vi "剔除拟合空白数据.vi"(2 "输入数组 2":dbl[](array[numeric])=[6.403, 7.477, 8.047, 8.638, 10.5185], 3 "输入数组":dbl[](array[numeric])=[6.403, 7.477, 8.047, 8.638, 10.5185]) -> (0 "输出数组 2":dbl[](array[numeric])=[6.403, 7.477, 8.047, 8.638, 10.5185], 1 "输出数组":dbl[](array[numeric])=[6.403, 7.477, 8.047, 8.638, 10.5185])   [LabVIEW 2014]
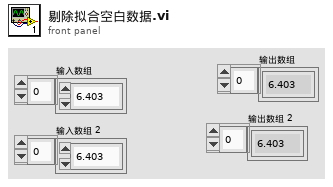
[diagram p1: front panel]
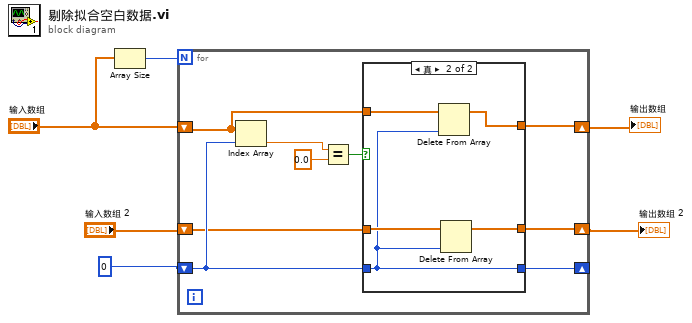
[diagram p0: block diagram]
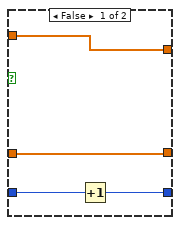
[diagram p2: hidden frame]
diagram:
  n1 = Array Size(array="输入数组") -> (size(s)=w2:i32)
  n2 = for {
    N: w2 -> [_]
    shift-right: [w7] -> w5
    shift-left: "输入数组 2" -> [w8]
    shift-right: [w9] -> _
    shift-left: 0 -> [w11]
    shift-right: [w10] -> w3
    shift-left: "输入数组" -> [w12]
    n3 = Index Array(array=w12, index=w11) -> (element=w13:dbl)
    n4 = Equal?(x=w13, y=0.0) -> (x = y?=w15:bool)
    n5 = case shown="真" w15 {
      tunnel: w12 -> [w19 w24]
      tunnel: [w19 w23] -> w10
      tunnel: w11 -> [w17 w20]
      tunnel: [w16 w20] -> w9
      tunnel: w8 -> [w18 w22]
      tunnel: [w18 w21] -> w7
      frame False {
        n6 = Increment(x=w17) -> (x+1=w16:i32)
      }
      frame True {
        n7 = Delete From Array(array=w24, index=w20) -> (array with subset deleted=w23:dbl[])  [unwired: 1 in, 1 out]
        n8 = Delete From Array(array=w22, index=w20) -> (array with subset deleted=w21:dbl[])  [unwired: 1 in, 1 out]
      }
    }
  }
  "输出数组" <- w3
  "输出数组 2" <- w5
